vi "MainGUI.vi"(8 "ErrorIn":errorcluster, 11 "YAFFooter:YAFFooter in":refnum<class "YAFFooter.lvclass">) -> ()   [LabVIEW 2021, in "YAFFooter.lvlib" / "YAFFooter.lvclass"]
doc: "This is the user interface of the object. It will handle the events to update the GUI."
uses:
  YAFFooter.lvclass
  C:/Localdata/Projects/TriekselSoft/TriekselsoftApplicationFramework/Source/.Externals/Library_YAF/YActor/YActor.lvclass
  YAFFooter.lvclass/YAFFooter.ctl
  YAFFooter_UiCallBackEvents.ctl
  YAFFooter_ClassCast.vi
  .Externals/Library_TAF/YActor/YActor.lvclass
panel:
  in  "Error":bool
  out "String":string
  out "L_busy":i32
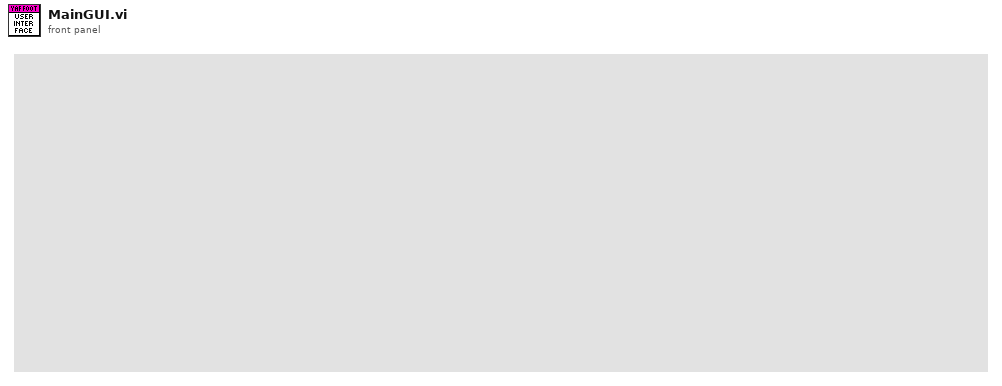
[diagram p1: front panel]
types:
  T1 = enum8{"Enabled", "Disabled", "Disabled and Grayed Out"}
  T2 = typedef "YAFFooter.lvlib/YAFFooter.lvclass/YAFFooter_UiCallBackEvents.ctl" = enum16{"Default", "PersistentDataUpdated"}
  T3 = cluster{"Event":string, "This":refnum<class>, "Data":variant}
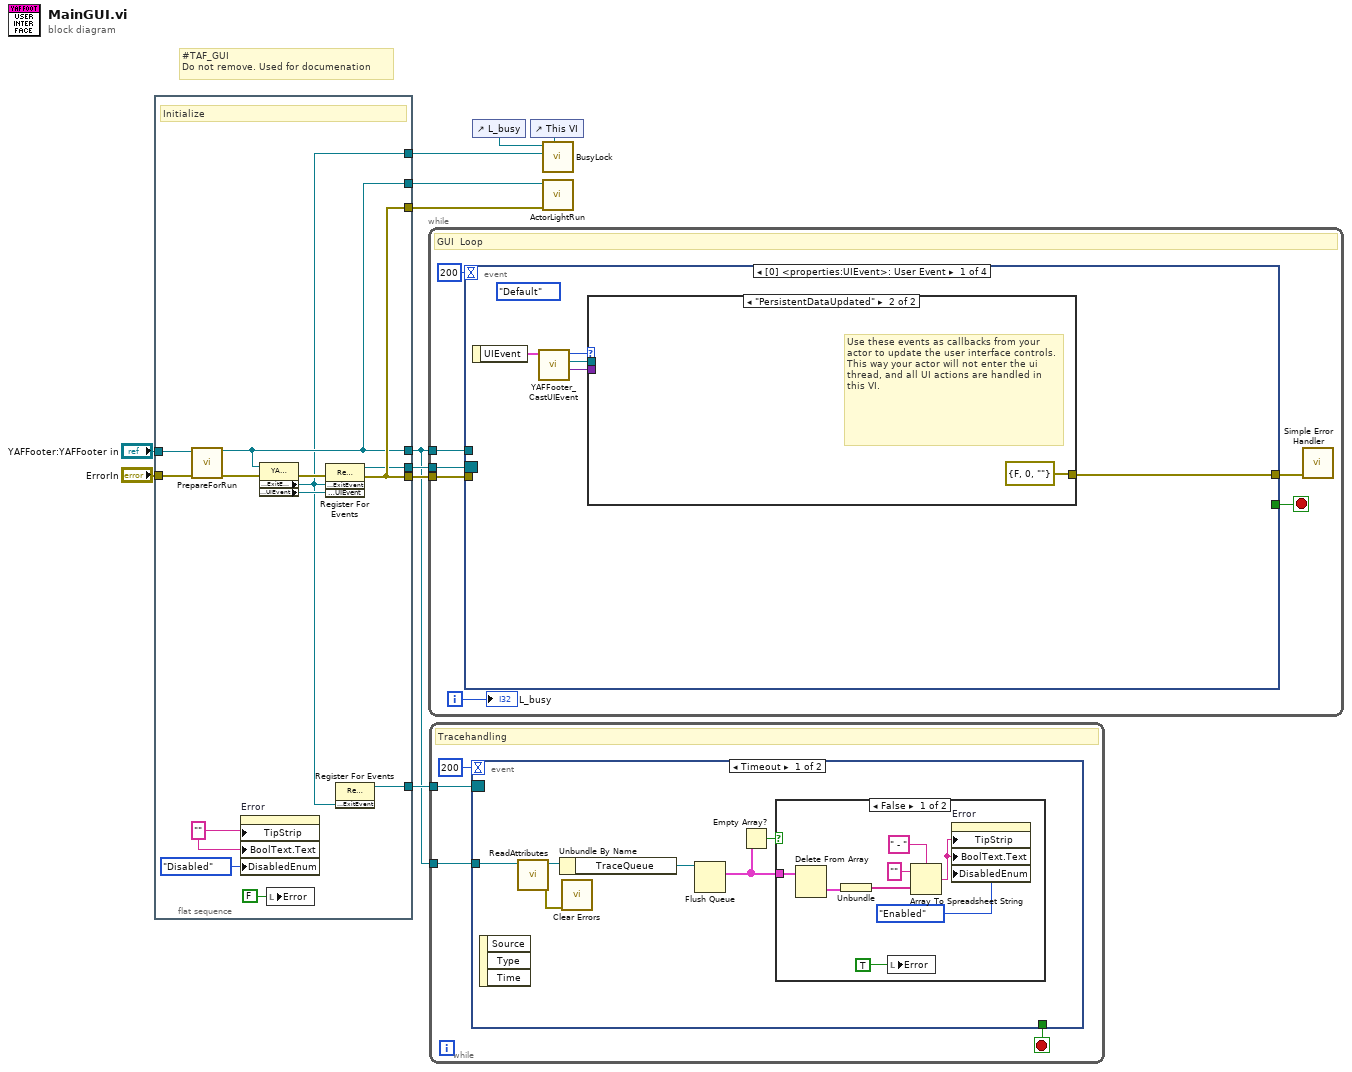
[diagram p0: block diagram]
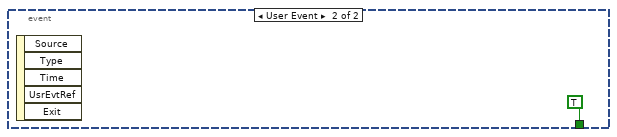
[diagram p3: hidden frame]
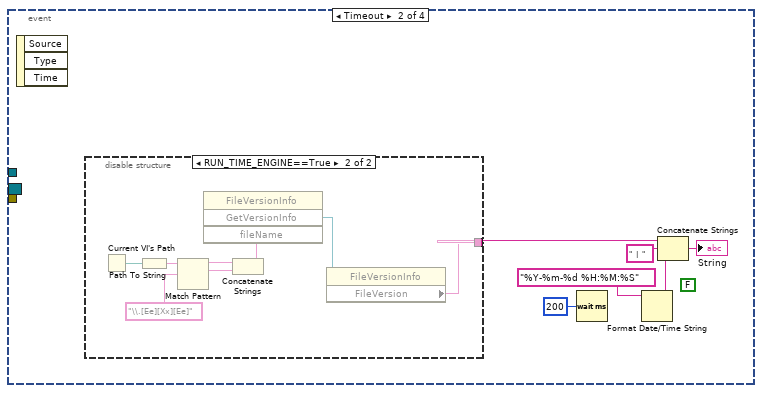
[diagram p5: hidden frame]
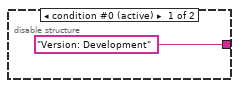
[diagram p6: hidden frame]
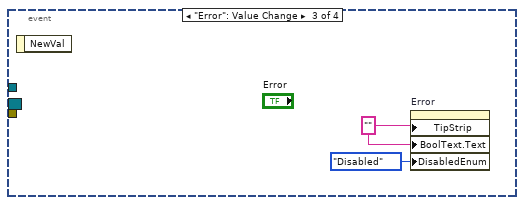
[diagram p7: hidden frame]
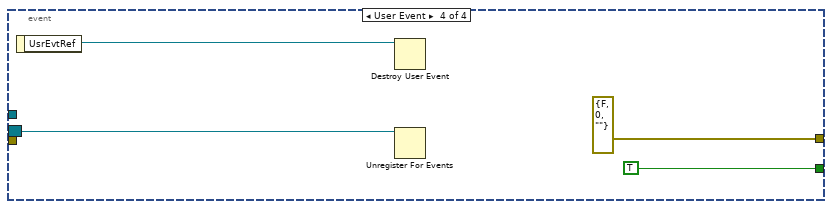
[diagram p8: hidden frame]
diagram:
  # "#TAF_GUI\nDo not remove. Used for documenation"
  n1 = flat-sequence {
    tunnel: "ErrorIn" -> [w24]
    tunnel: "YAFFooter:YAFFooter in" -> [w20]
    tunnel: [w19] -> w7
    tunnel: [w16] -> w4
    tunnel: [w18] -> w1
    tunnel: [w21] -> w10
    tunnel: [w18] -> w3
    tunnel: [w21] -> w9
    tunnel: [w15] -> w2
    frame #0 {
      w12 = "" ("Tip Strip")
      # "Initialize"
      n2 = call-dynamic "PrepareForRun.vi"("ErrorIn"=w24, "YActorIn"=w20) -> ("ErrorOut"=w22:errorcluster, "YActorOut"=w18:refnum<class "YAFFooter.lvclass">)  [unwired: 8 in]
      n3 = property on="Error" class="Bool (strict)"("TipStrip"=w12, "BoolText.Text"=w12, "DisabledEnum"=T1."Disabled" ("Disabled")) -> ()  [unwired: 2 in, 2 out]
      n4 = property class="YAFFooter"(reference=w18, error in=w22) -> (error out=w23:errorcluster, "properties:ExitEvent"=w16:refnum<user-event>, "properties:UIEvent"=w17:refnum<user-event>)  [unwired: 1 out]
      n5 = local write "Error"(FALSE ("Error")) -> ()
      n6 = register-events(error in=w23, w16, w17) -> (reference out=w19:refnum<event-registration>, error out=w21:errorcluster)  [unwired: 1 in]
      n7 = register-events(w16) -> (reference out=w15:refnum<event-registration>)  [unwired: 2 in, 1 out]
    }
  }
  n8 = while {
    tunnel: w10 -> [w31]
    tunnel: w7 -> [w28]
    tunnel: w1 -> [w25]
    i -> [w27]
    stop <- w29 stop-if-true
    # "GUI  Loop"
    n9 = event shown="[0] <properties:UIEvent>: User Event" {
      selector: w28 -> [_ _ _ w56]
      dyn-events: _ -> [_ _ _ _]
      timeout: 200 -> [_ _ _ _]
      tunnel: w31 -> [_ _ _ _]
      tunnel: [_ _ _ TRUE] -> w29
      tunnel: [w36 _ _ errorcluster {"status"=FALSE, "code"=0, "source"=""} ("error constant")] -> w30
      tunnel: w25 -> [_ _ _ _]
      event User Event {
        (unwired) YAFFooter_UiCallBackEvents."Default" ("UiEventNames")
        n10 = event-data() -> ("UIEvent"=w35:T3)  [unwired: 1 in]
        n11 = call "YAFFooter_CastUIEvent.vi"("UIEvent"=w35) -> ("Data"=w32:variant, "ApplicationGUIOut"=w33:refnum<class "YAFFooter.lvclass">, "UiEventNames"=w34:T2)  [unwired: 8 in]
        n12 = case shown="\"PersistentDataUpdated\"" w34 {
          tunnel: w33 -> [_ _]
          tunnel: w32 -> [_ _]
          tunnel: [_ errorcluster {"status"=FALSE, "code"=0, "source"=""} ("ErrorOut")] -> w36
          frame Default {
          }
          frame "PersistentDataUpdated" {
            # "Use these events as callbacks from your actor to update the user interface controls. This way your actor will not enter the ui thread, and all UI actions are handled in this VI."
          }
        }
      }
      event Timeout {
        (unwired) FALSE
        n13 = event-data() -> ()  [unwired: 1 in, 3 out]
        n14 = disable-structure shown="RUN_TIME_ENGINE==True" {
          disable-tunnel: ["Version: Development" w45] -> w43
          frame condition #0 (active) {
          }
          frame condition #1 {
            n15 = Current VI's Path() -> (path=w48:path)
            n16 = Path To String(path=w48) -> (string=w52:string)
            n17 = Match Pattern(string=w52, regular expression="\\.[Ee][Xx][Ee]") -> (before substring=w50:string, match substring=w49:string)  [unwired: 1 in, 2 out]
            n18 = Concatenate Strings(w50, w49) -> (w51:string)
            n19 = invoke class="FileVersionInfo" method="GetVersionInfo"("fileName"=w51) -> ("GetVersionInfo"=w47:refnum<k24>)  [unwired: 3 in, 3 out]
            n20 = property class="FileVersionInfo"(reference=w47) -> ("FileVersion"=w45:string)  [unwired: 1 in, 2 out]
          }
        }
        n21 = Wait (ms)(milliseconds to wait=u32 200) -> ()  [unwired: 1 out]
        n22 = Format Date/Time String(time format string (%c)="%Y-%m-%d %H:%M:%S") -> (date/time string=w40:string)  [unwired: 2 in]
        n23 = Concatenate Strings(w43, "  |  " ("string"), w40) -> (→"String":string)
      }
      event "Error": Value Change {
        w54 = "" ("Tip Strip")
        n24 = event-data() -> ()  [unwired: 1 in, 1 out]
        n25 = property on="Error" class="Bool (strict)"("TipStrip"=w54, "BoolText.Text"=w54, "DisabledEnum"=T1."Disabled" ("Disabled")) -> ()  [unwired: 2 in, 2 out]
      }
      event User Event {
        n26 = event-data() -> ("UsrEvtRef"=w55:refnum<user-event>)  [unwired: 1 in]
        n27 = Destroy User Event(user event=w55) -> ()  [unwired: 1 in, 1 out]
        n28 = Unregister For Events(event registration refnum=w56) -> ()  [unwired: 1 in, 1 out]
      }
    }
    n29 = call <vilib>:"Simple Error Handler.vi"("error in (no error)"=w30) -> ()  [unwired: 4 in, 5 out]
    "L_busy" <- w27
  }
  n30 = while {
    tunnel: w2 -> [w62]
    tunnel: w1 -> [w59]
    stop <- w61 stop-if-true
    # "Tracehandling"
    n31 = event shown="[0] Timeout" {
      selector: w62 -> [_ _]
      dyn-events: _ -> [_ _]
      timeout: 200 -> [_ _]
      tunnel: [_ TRUE] -> w61
      tunnel: w59 -> [w64 _]
      event Timeout {
        n32 = event-data() -> ()  [unwired: 1 in, 3 out]
        n33 = call "ReadAttributes.vi"("YActorIn"=w64) -> ("ErrorOut"=w63:errorcluster, "YActorOut"=w65:refnum<class "YAFFooter.lvclass">)  [unwired: 9 in]
        n34 = Unbundle By Name(w65) -> ("TraceQueue"=w66:refnum<queue>)
        n35 = call <vilib>:"Clear Errors.vi"("error in (no error)"=w63) -> ()  [unwired: 5 in, 2 out]
        n36 = Flush Queue(queue=w66) -> (remaining elements=w68:cluster{string[]}[])  [unwired: 1 in, 2 out]
        n37 = Empty Array?(array=w68) -> (empty?=w67:bool)
        n38 = case shown="False" w67 {
          tunnel: w68 -> [w76 _]
          frame False {
            n39 = Delete From Array(array=w76) -> (deleted portion=w72:cluster{string[]})  [unwired: 2 in, 1 out]
            n40 = Unbundle(w72) -> (w73:string[])
            n41 = local write "Error"(TRUE ("Error")) -> ()
            n42 = Array To Spreadsheet String(delimiter (Tab)=" - ", array=w73, 3:"" ("format string")) -> (spreadsheet string=w71:string)
            n43 = property on="Error" class="Bool (strict)"("TipStrip"=w71, "BoolText.Text"=w71, "DisabledEnum"=T1."Enabled" ("Disabled")) -> ()  [unwired: 2 in, 2 out]
          }
          frame True {
          }
        }
      }
      event User Event {
        n44 = event-data() -> ()  [unwired: 1 in, 5 out]
      }
    }
  }
  n45 = control-ref of="L_busy"() -> (w6:refnum<vi>)
  n46 = control-ref of="This VI"() -> (w5:refnum<vi>)
  n47 = call "BusyLock.vi"("BusyLock"=w5, "ExitEvent"=w4, "Counter"=w6) -> ()  [unwired: 9 in]
  n48 = call "ActorLightRun.vi"("ErrorIn"=w9, "YActorIn"=w3) -> ()  [unwired: 8 in, 2 out]
